vi "Write Output.vi"(8 "error in (no error)":errorcluster, 10 "output":dbl, 11 "PID Loop in":refnum<class "PID Loop.lvclass">) -> (0 "error out":errorcluster, 3 "PID Loop out":refnum<class "PID Loop.lvclass">)   [LabVIEW 2024, in "PID Loop.lvlib" / "PID Loop.lvclass"]
uses:
  PID Loop.lvclass
  PID Loop.lvclass/PID Loop.ctl
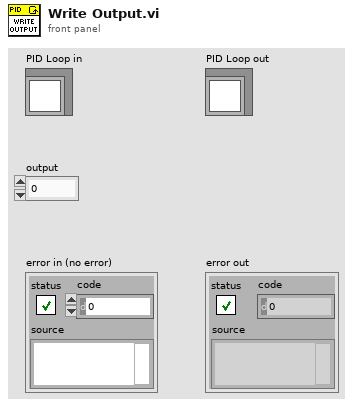
[diagram p1: front panel]
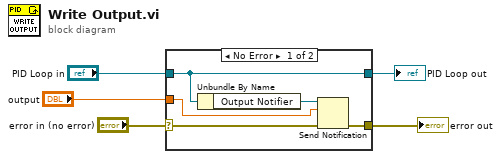
[diagram p0: block diagram]
diagram:
  n1 = case shown="No Error" "error in (no error)" {
    selector: "error in (no error)" -> [w7 w12]
    tunnel: [w6 w12] -> w4
    tunnel: [w10 w11] -> w2
    tunnel: "PID Loop in" -> [w10 w11]
    tunnel: "output" -> [w8 _]
    frame No Error {
      n2 = Unbundle By Name(w10) -> ("Output Notifier"=w9:refnum<notifier>)
      n3 = Send Notification(notification=w8, notifier=w9, error in (no error)=w7) -> (error out=w6:errorcluster)  [unwired: 1 out]
    }
    frame Error {
    }
  }
  "error out" <- w4
  "PID Loop out" <- w2
